vi "MultipleLines to String.vi"(11 "Array":string[](array[string])) -> (3 "String":string)   [LabVIEW 2017, in "LabVIEW-Config.lvlib" / "LabVIEW-Config.lvclass"]
uses:
  LabVIEW-Config.lvclass
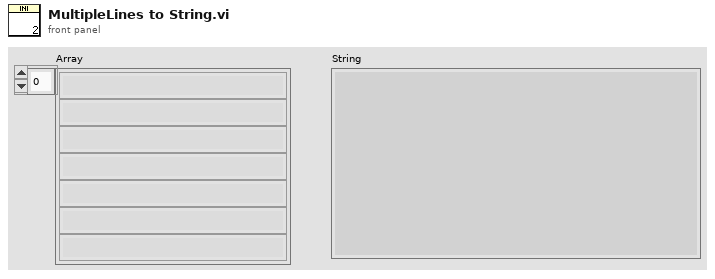
[diagram p1: front panel]
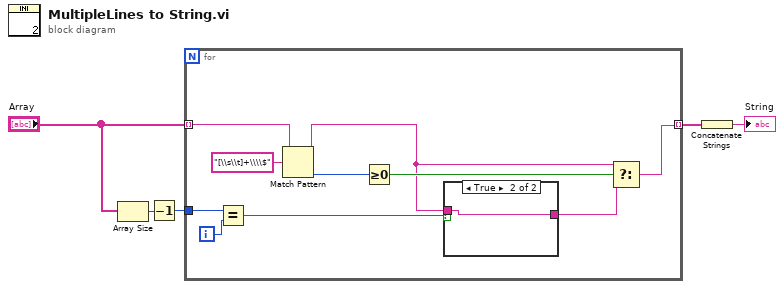
[diagram p0: block diagram]
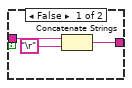
[diagram p2: hidden frame]
diagram:
  n1 = Array Size(array="Array") -> (size(s)=w2:i32)
  n2 = Decrement(x=w2) -> (x-1=w1:i32)
  n3 = for {
    tunnel: "Array" -> [w15] mode=indexing
    tunnel: [w9] -> w4 mode=indexing
    tunnel: w1 -> [w8]
    i -> [w7]
    n4 = Equal?(x=w8, y=w7) -> (x = y?=w6:bool)
    n5 = Match Pattern(string=w15, regular expression="[\\s\\t]+\\\\$") -> (before substring=w11:string, offset past match=w13:i32)  [unwired: 1 in, 2 out]
    n6 = Greater Or Equal To 0?(x=w13) -> (x >= 0?=w12:bool)
    n7 = case shown="True" w6 {
      tunnel: w11 -> [w18 w19]
      tunnel: [w17 w19] -> w10
      frame False {
        n8 = Concatenate Strings(w18, "\r") -> (w17:string)
      }
      frame True {
      }
    }
    n9 = Select(t=w11, s=w12, f=w10) -> (s? t:f=w9:string)
  }
  n10 = Concatenate Strings(w4) -> (→"String":string)
